vi "CheckLimStat.vi"(3 "Always Warn?":bool, 4 "# Axis":i8=1, 5 "Motion Board ID":u8 min=1 max=32 step=1) -> ()   [LabVIEW 2022 SP3]
uses:
  -MotionRoutines/MotionGlobals.vi
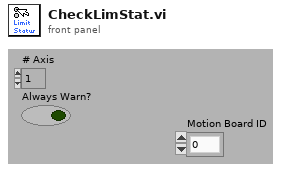
[diagram p1: front panel]
types:
  T1 = typedef "Axis Status (8 axes).flx" = cluster{"1":bool, "2":bool, "3":bool, "4":bool, "5":bool, "6":bool, "7":bool, "8":bool}
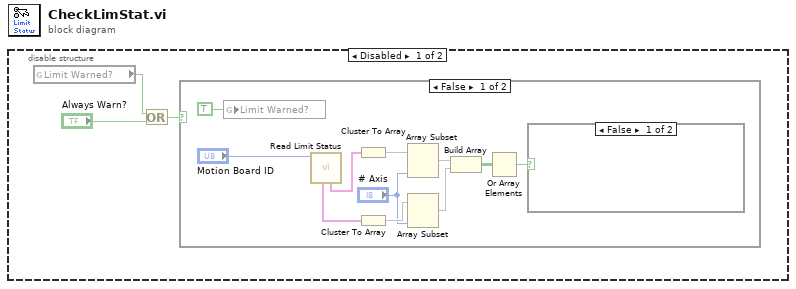
[diagram p0: block diagram]
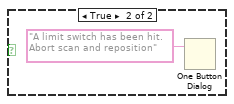
[diagram p2: hidden frame]
diagram:
  n1 = disable-structure shown="Disabled" {
    frame Disabled {
      n2 = global read "MotionGlobals.vi" "Limit Warned?"() -> (w3:bool)
      n3 = Or(x=w3, y="Always Warn?") -> (x .or. y?=w2:bool)
      n4 = case shown="False" w2 {
        frame False {
          n5 = global write "MotionGlobals.vi" "Limit Warned?"(TRUE ("Limit Warned?")) -> ()
          n6 = call <vilib>:"Read Limit Status.vi"("Board ID"="Motion Board ID") -> ("Reverse Limits"=w12:T1, "Forward Limits"=w13:T1)  [unwired: 7 in, 2 out]
          n7 = Cluster To Array(cluster=w12) -> (array=w11:bool[])
          n8 = Cluster To Array(cluster=w13) -> (array=w9:bool[])
          n9 = Array Subset(array=w11, length="# Axis") -> (w10:bool[])  [unwired: 1 in]
          n10 = Array Subset(array=w9, length="# Axis") -> (w6:bool[])  [unwired: 1 in]
          n11 = Build Array(w10, w6) -> (w7:bool[][])
          n12 = Or Array Elements(Boolean array=w7) -> (logical OR=w5:bool)
          n13 = case shown="False" w5 {
            frame False {
            }
            frame True {
              n14 = One Button Dialog(message="A limit switch has been hit. Abort scan and reposition") -> ()  [unwired: 1 in, 1 out]
            }
          }
        }
        frame True {
        }
      }
    }
    frame Enabled {
    }
  }
